vi "Ticks To Radians.vi"(1 "Ticks/Rev":i32=4096, 2 "Ticks":dbl) -> (0 "Radians":dbl)   [LabVIEW 2016, in "Huskie Swerve.lvlib"]
uses:
  Huskie Swerve.lvlib
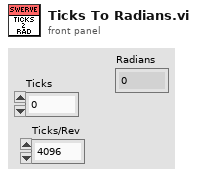
[diagram p1: front panel]
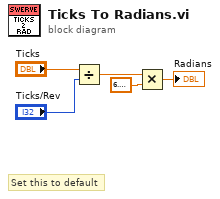
[diagram p0: block diagram]
diagram:
  # "Set this to default"
  n1 = Divide(x="Ticks", y="Ticks/Rev") -> (x/y=w4:dbl)
  n2 = Multiply(x=w4, y=6.283185307179586) -> (x*y=→"Radians":dbl)
